vi "Rename Device Dialog.vi"(8 "error in (no error)":errorcluster, 9 "new device name":string, 10 "old device name":string) -> (0 "error out":errorcluster, 1 "new device name out":string="NI-SLSC-30BE717f", 2 "old device name out":string="NI-SLSC-30BE717e", 3 "Cancelled?":bool)   [LabVIEW 2017]
doc: "Use this template to create a dialog box with event handling."
panel:
  in  "Cancel":bool
  in  "OK":bool=TRUE
  # "Old Device Name"
  # "New Device Name"
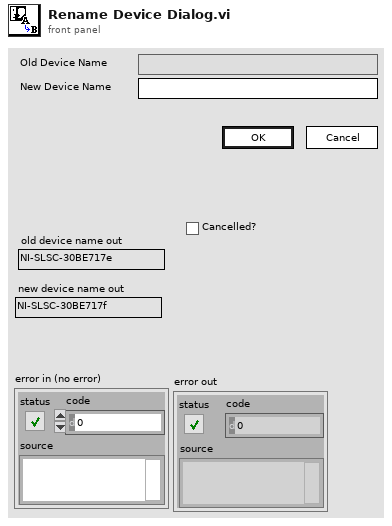
[diagram p1: front panel]
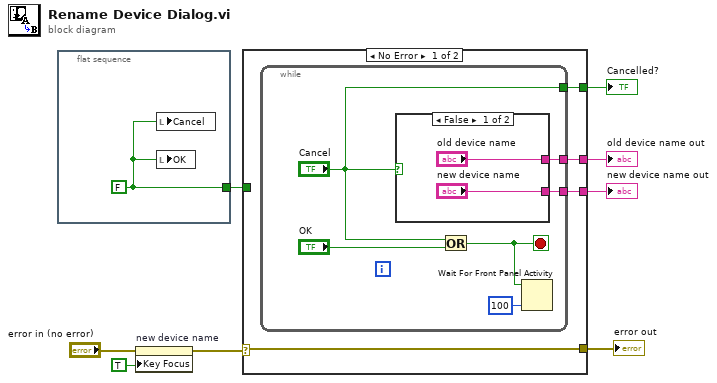
[diagram p0: block diagram]
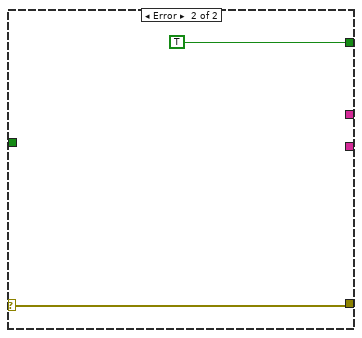
[diagram p3: hidden frame]
diagram:
  n1 = flat-sequence {
    tunnel: [w9] -> w4
    frame #0 {
      w9 = FALSE
      n2 = local write "Cancel"(w9) -> ()
      n3 = local write "OK"(w9) -> ()
    }
  }
  n4 = property on="new device name" class="Str"(error in="error in (no error)", "Key Focus"=TRUE) -> (error out=w3:errorcluster)  [unwired: 1 in, 1 out]
  n5 = case shown="No Error" w3 {
    selector: w3 -> [w10 w23]
    tunnel: [w13 TRUE ("Cancel")] -> w8
    tunnel: [w12 _] -> w7
    tunnel: [w11 _] -> w6
    tunnel: [w10 w23] -> w5
    tunnel: w4 -> [_ _]
    frame No Error {
      n6 = while {
        tunnel: ["Cancel"] -> w13
        tunnel: [w18] -> w12
        tunnel: [w16] -> w11
        stop <- w15 stop-if-true
        n7 = case shown="False" "Cancel" {
          tunnel: ["old device name" _] -> w18
          tunnel: ["new device name" _] -> w16
          frame False {
          }
          frame True {
          }
        }
        n8 = Or(x="Cancel", y="OK") -> (x .or. y?=w15:bool)
        n9 = Wait For Front Panel Activity(1:100 ("timeout ms (-1 never timeout)"), 3:w15) -> ()  [unwired: 1 in, 1 out]
      }
    }
    frame Error {
    }
  }
  "Cancelled?" <- w8
  "old device name out" <- w7
  "new device name out" <- w6
  "error out" <- w5
